vi "Create Map.vi"() -> ()   [LabVIEW 2016, in "Map.lvclass"]
uses:
  Map.lvclass
  Grid/Grid.lvclass
panel:
  in  "Map.lvclass":refnum<class "Map.lvclass">
  out "Value":picture
  out "Array":picture[][](array[picture])
  in  "Iterations":u16
  out "Numeric 2":i32
  out "Numeric":i32
  in  "Map":T1={"Width"=250, "Height"=250, "Iterations"=256, "Top Left Coordinate"=-2.5+1.0i, "Bottom Right Coordinate"=1.0-1.0i}
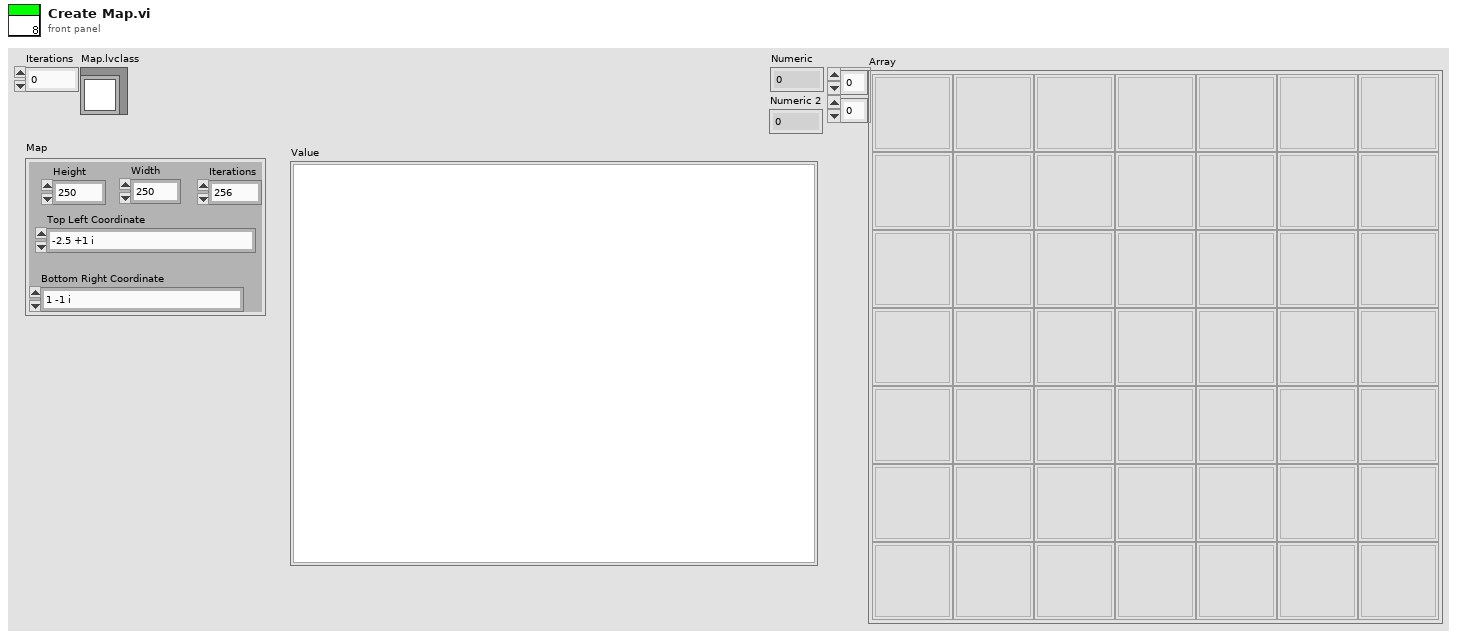
[diagram p1: front panel]
types:
  T1 = cluster{"Width":i32, "Height":i32, "Iterations":u16, "Top Left Coordinate":cdb, "Bottom Right Coordinate":cdb}
  T2 = cluster{"Width":i32, "Height":i32, "Iterations":u16, "Top Left Coordinate":cdb, "Bottom Right Coordinate":cdb}[][]
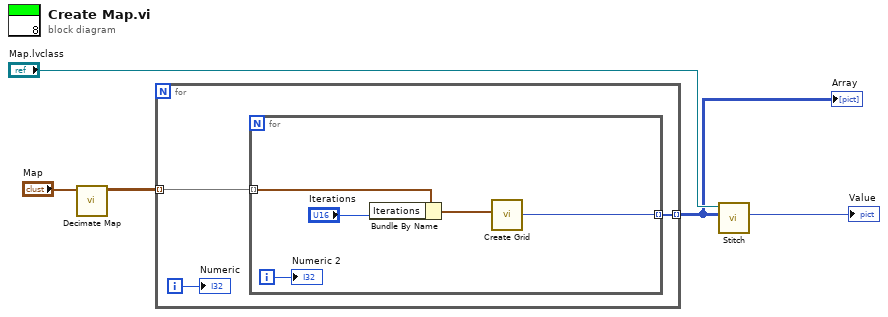
[diagram p0: block diagram]
diagram:
  n1 = call "Decimate Map.vi"("Map"="Map") -> ("Decimated Map"=w4:T2)  [unwired: 10 in]
  n2 = for {
    tunnel: w4 -> [w8] mode=indexing
    tunnel: [w6] -> w1 mode=indexing
    i -> [w7]
    n3 = for {
      tunnel: w8 -> [w12] mode=indexing
      tunnel: [w9] -> w6 mode=indexing
      i -> [w13]
      n4 = Bundle By Name(cluster=w12, "Iterations"="Iterations") -> (w10:T1)
      n5 = call "Create Grid.vi"("input cluster"=w10) -> ("new picture"=w9:picture)  [unwired: 9 in, 1 out]
      "Numeric 2" <- w13
    }
    "Numeric" <- w7
  }
  "Array" <- w1
  n6 = call "Stitch.vi"("Array"=w1, "Map.lvclass"="Map.lvclass") -> ("Value"=→"Value":picture)  [unwired: 8 in, 1 out]
